vi "Read U8 Array.vi"(7 "Channel Array in":refnum<class "CIFChannels.lvclass">[](array[class]), 8 "error in (no error)":errorcluster, 10 "Channel Index":i32) -> (0 "error out":errorcluster, 1 "timed out?":bool, 2 "Data":u8[](array[numeric]), 4 "Header":T1, 5 "Channel Array out":refnum<class "CIFChannels.lvclass">[](array[class]))   [LabVIEW 2021, in "CIFChannelMng.lvclass"]
uses:
  CIFChannelMng.lvclass
  <vilib>/CIF Foundation/CIF Channels Core/ChannelCommon/typedef/FIFO Header.ctl
  CIFChannelMng.lvclass/CIFChannelMng.ctl
  <vilib>/CIF Foundation/CIF Channels Core/CIFChannels/CIFChannels.lvclass
  <vilib>/CIF Foundation/CIF Channels Core/ChannelCommon/ChannelCommon.lvlib
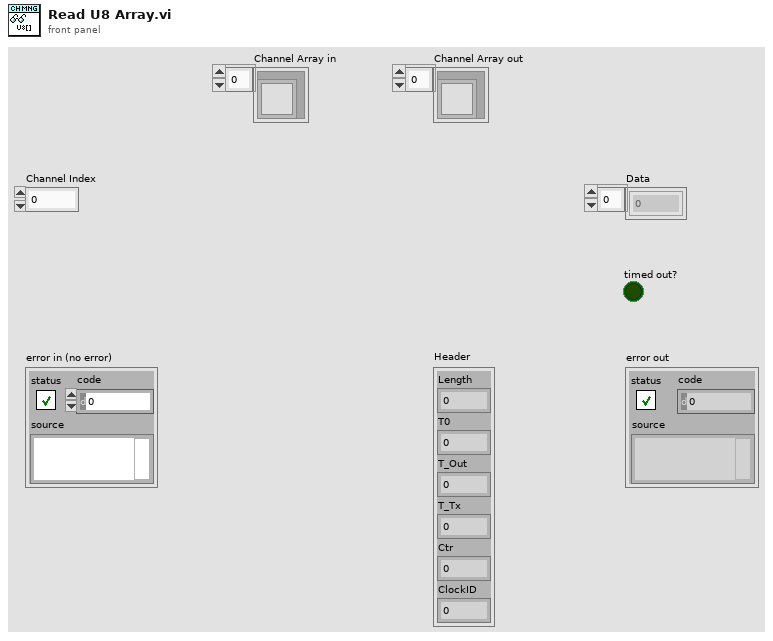
[diagram p1: front panel]
types:
  T1 = typedef "ChannelCommon.lvlib/FIFO Header.ctl" = cluster{"Length":u64, "T0":i64, "T_Out":i64, "T_Tx":i64, "Ctr":u64, "ClockID":u8}
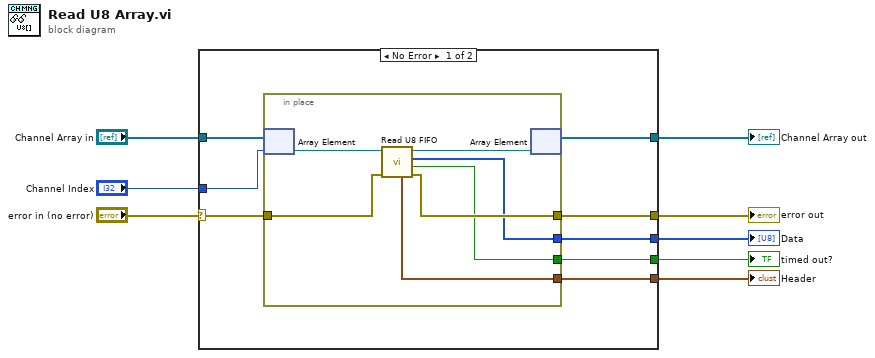
[diagram p0: block diagram]
diagram:
  n1 = case shown="No Error" "error in (no error)" {
    selector: "error in (no error)" -> [w16 w25]
    tunnel: [w15 w25] -> w7
    tunnel: [w9 w24] -> w1
    tunnel: "Channel Array in" -> [w10 w24]
    tunnel: [w14 _] -> w4
    tunnel: [w13 _] -> w6
    tunnel: "Channel Index" -> [w12 _]
    tunnel: [w11 _] -> w3
    frame No Error {
      n2 = in-place {
        in-place-border: w16 -> [w23]
        in-place-border: [w22] -> w15
        in-place-border: [w21] -> w13
        in-place-border: [w20] -> w14
        in-place-border: [w17] -> w11
        n3 = in-place-array #1(w10, w12) -> (w19:refnum<class "CIFChannels.lvclass">)
        n4 = call-dynamic "Read U8 FIFO.vi"("error in (no error)"=w23, "CIFChannels in"=w19) -> ("error out"=w22:errorcluster, "timed out?"=w21:bool, "Data out"=w20:u8[], "CIFChannels out"=w18:refnum<class "CIFChannels.lvclass">, "Header"=w17:T1)  [unwired: 5 in]
        n5 = in-place-array #1(w18) -> (w9:refnum<class "CIFChannels.lvclass">[])  [unwired: 1 out]
      }
    }
    frame Error {
    }
  }
  "error out" <- w7
  "timed out?" <- w6
  "Data" <- w4
  "Header" <- w3
  "Channel Array out" <- w1
